vi "Write Result.vi"(8 "error in (no error)":errorcluster, 10 "Result":dbl, 11 "Controller in":refnum<class "Controller.lvclass">) -> (0 "error out":errorcluster, 3 "Controller out":refnum<class "Controller.lvclass">)   [LabVIEW 2013, in "Controller.lvlib" / "Controller.lvclass"]
uses:
  Controller.lvclass
  Controller.lvclass/Controller.ctl
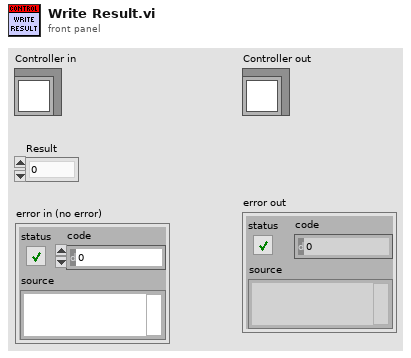
[diagram p1: front panel]
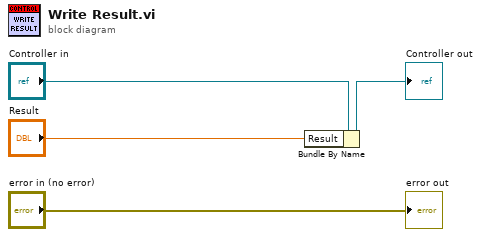
[diagram p0: block diagram]
diagram:
  n1 = Bundle By Name(cluster="Controller in", "Result"="Result") -> (→"Controller out":refnum<class "Controller.lvclass">)
  "error out" <- "error in (no error)"
